vi "Rcv Cmd.vi"(8 "error in":errorcluster, 11 "nPAS in":refnum<class "nPAS.lvclass">) -> (0 "error out":errorcluster, 3 "nPAS out":refnum<class "nPAS.lvclass">)   [LabVIEW 2015, in "nPAS.lvclass"]
doc: "This function is abstract and the child must overide it. This function should provide a means by which the user may interact with the PAS."
uses:
  nPAS.lvclass
  Session/Raw FPGA/FPGA Session.lvclass
  nPAS.lvclass/nPAS.ctl
  Session/Raw FPGA/FPGA Session.lvclass/FPGA Session.ctl
  FPGA/fpga dio enum.ctl
  Reusable/PAS/Main/PAS.lvclass/PAS.ctl
  Reusable/Instrument/state.ctl
  Reusable/PAS/Main/Write Chirp.vi
  Session/Raw FPGA/Read FPGA Ref.vi
  <vilib>/Utility/error.llb/Error Cluster From Error Code.vi
  <vilib>/rvi/errors/niLvFpgaAdjustHostInterfaceError.vi
  Reusable/PAS/Main/Set Speaker Switch.vi
  FPGA Ref.ctl
  <vilib>/rvi/interface/nirviReadWriteControl/nirviReadWriteControl.xnode
  FPGA Bitfiles/NickIO.lvbitx
  <vilib>/rvi/interface/nirviMethod/nirviMethod.xnode
  FPGA/PAS Modulation.ctl
  Reusable/Instrument/Instrument.lvclass
  NiFpgaLv.dll
  <vilib>/rvi/errors/niLvFpgaMergeErrorWithErrorCode.vi
  <vilib>/FPGAPlugInAG/cRIO-9081/niLvFpga_WriteFifo_cRIO-9081.vi
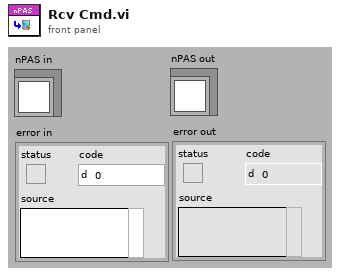
[diagram p1: front panel]
types:
  T1 = typedef "fpga dio enum.ctl" = enum16{"uv.ctl_1", "uv.ctl_2", "uv.enable", "pas.las_enable", "pas.speaker", "compressor", "vacuum", "sol.o3_add", "sol.scubber_test", "sol.pmeas1", "sol.pmeas2", "filt.hb_ctl_1", "filt.hb_ctl_2", "crd.las_enable"}
  T2 = typedef "Instrument.lvclass/state.ctl" = enum8{"Configure", "Acquire", "Wait", "Quit", "Handle Error", "NOOP"}
  T3 = typedef "Session - Root.lvclass/Session Handle.ctl" = refnum<data-value>
  T4 = typedef "FPGA Ref.ctl" = refnum<k20>
  T5 = cluster{"Array of Int16[0]":i16, "Array of Int16[1]":i16}
  T6 = typedef "PAS Modulation.ctl" = cluster{"f0":fxp<+,32,0>, "Mod":u8, "Vscale":fxp<+,32,0>, "Offset":i16}
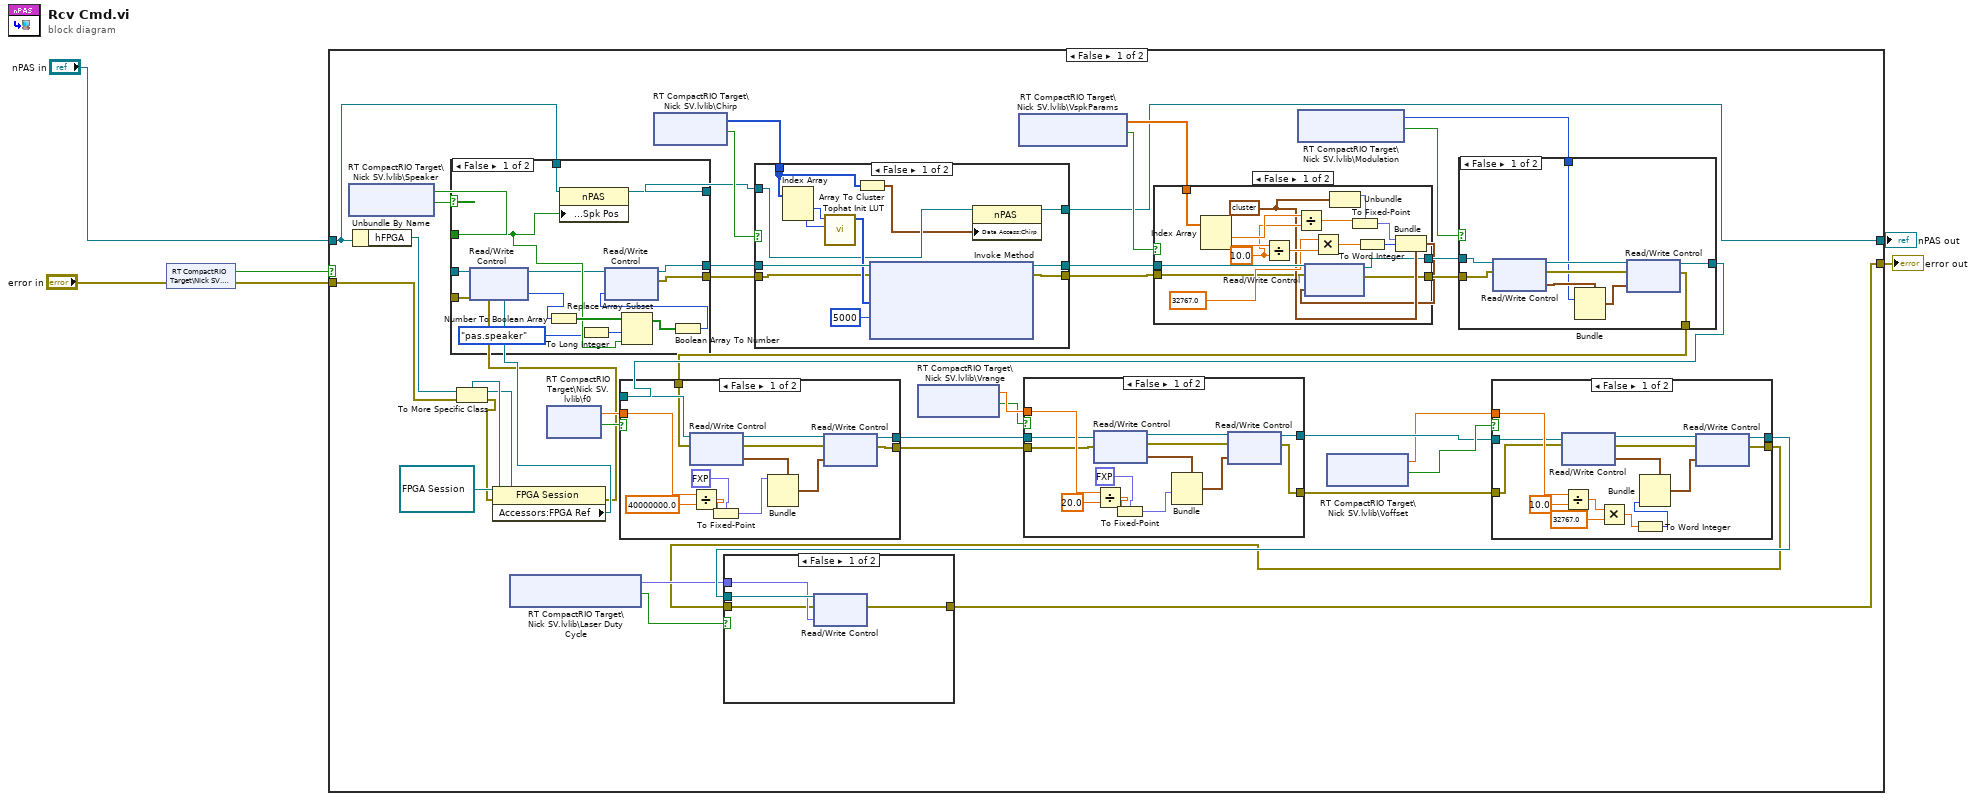
[diagram p0: block diagram]
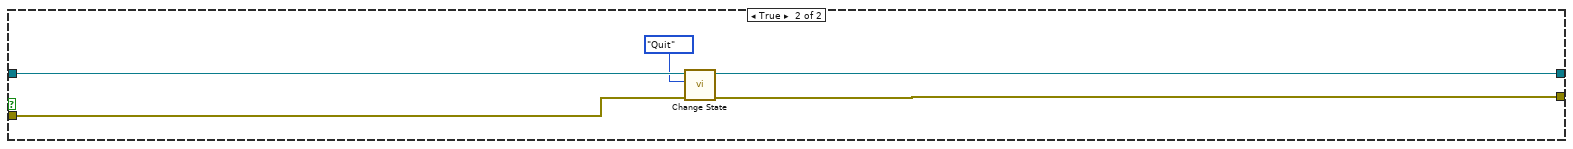
[diagram p10: hidden frame]
diagram:
  n1 = shared-variable "RT CompactRIO Target\\Nick SV.lvlib\\Stop"(error in="error in") -> (w5:bool, error out=w2:errorcluster)
  n2 = case shown="False" w5 {
    tunnel: "nPAS in" -> [w9 w165]
    tunnel: [w7 w164] -> w3
    tunnel: w2 -> [w14 w162]
    tunnel: [w18 w161] -> w1
    frame False {
      n3 = shared-variable "RT CompactRIO Target\\Nick SV.lvlib\\Speaker"() -> (w46:bool, w47:bool)  [unwired: 2 in, 1 out]
      n4 = Unbundle By Name(w9) -> ("hFPGA"=w16:T3)
      n5 = To More Specific Class(target class=refnum<data-value> refnum ("hFPGA"), reference=w16, error in=w14) -> (specific class reference=w13:refnum<data-value>, error out=w12:errorcluster)
      n6 = property class="FPGA Session"(reference=w13, error in=w12) -> (error out=w10:errorcluster, "Accessors:FPGA Ref"=w11:T4)  [unwired: 1 out]
      n7 = case shown="False" w47 {
        tunnel: w46 -> [w149 _]
        tunnel: w11 -> [w153 w160]
        tunnel: [w157 w160] -> w43
        tunnel: [w156 w159] -> w28
        tunnel: w10 -> [w152 w159]
        tunnel: w9 -> [w155 w158]
        tunnel: [w154 w158] -> w8
        frame False {
          n8 = xnode "Read/Write Control"("FPGA VI Reference In"=w153, "error in"=w152) -> ("FPGA VI Reference Out"=w147:T4, "DO Out"=w151:u16)  [unwired: 1 out]
          n9 = Number To Boolean Array(number=w151) -> (Boolean array=w150:bool[])
          n10 = property class="nPAS"(reference=w155, "Data Access:Spk Pos"=w149) -> (reference out=w154:refnum<class "nPAS.lvclass">)  [unwired: 1 in, 1 out]
          n11 = To Long Integer(number=fpga_dio_enum."pas.speaker" ("fpga dio")) -> (32bit integer=w146:i32)
          n12 = Replace Array Subset(array=w150, new element=w149, index=w146) -> (w148:bool[])
          n13 = Boolean Array To Number(Boolean array=w148) -> (number=w144:u16)
          n14 = xnode "Read/Write Control"("FPGA VI Reference In"=w147, "DO In"=w144) -> ("FPGA VI Reference Out"=w157:T4, "error out"=w156:errorcluster)  [unwired: 1 in]
        }
        frame True {
        }
      }
      n15 = shared-variable "RT CompactRIO Target\\Nick SV.lvlib\\Laser Duty Cycle"() -> (w20:fxp<+,32,0>, w22:bool)  [unwired: 2 in, 1 out]
      n16 = shared-variable "RT CompactRIO Target\\Nick SV.lvlib\\f0"() -> (w35:dbl, w36:bool)  [unwired: 2 in, 1 out]
      n17 = shared-variable "RT CompactRIO Target\\Nick SV.lvlib\\Chirp"() -> (w44:i16[], w45:bool)  [unwired: 2 in, 1 out]
      n18 = case shown="False" w45 {
        tunnel: w44 -> [w130 _]
        tunnel: w43 -> [w138 w143]
        tunnel: [w135 w143] -> w41
        tunnel: w28 -> [w134 w142]
        tunnel: [w133 w142] -> w27
        tunnel: w8 -> [w132 w141]
        tunnel: [w131 w141] -> w7
        frame False {
          n19 = Index Array(array=w130) -> (element #1=w140:i16, element #2=w139:i16)  [unwired: 2 in]
          n20 = call "Tophat Init LUT.vi"("Df"=w139, "f0"=w140) -> ("Init Data Out"=w137:i16[])  [unwired: 7 in]
          n21 = Array To Cluster(array=w130) -> (cluster=w129:T5)
          n22 = xnode "Invoke Method"("FPGA VI Reference In"=w138, "error in"=w134, "Data"=w137, "Timeout (ms)"=5000) -> ("FPGA VI Reference Out"=w135:T4, "error out"=w133:errorcluster)  [unwired: 1 out]
          n23 = property class="nPAS"(reference=w132, "Data Access:Chirp"=w129) -> (reference out=w131:refnum<class "nPAS.lvclass">)  [unwired: 1 in, 1 out]
        }
        frame True {
        }
      }
      n24 = shared-variable "RT CompactRIO Target\\Nick SV.lvlib\\Vrange"() -> (w32:dbl, w17:bool)  [unwired: 2 in, 1 out]
      n25 = shared-variable "RT CompactRIO Target\\Nick SV.lvlib\\VspkParams"() -> (w40:sgl[], w42:bool)  [unwired: 2 in, 1 out]
      n26 = case shown="False" w42 {
        tunnel: w41 -> [w126 w128]
        tunnel: w40 -> [w125 _]
        tunnel: [w112 w128] -> w38
        tunnel: w27 -> [w111 w127]
        tunnel: [w110 w127] -> w26
        frame False {
          w119 = sgl 10.0 ("y")
          w116 = cluster{"Vscale":fxp<+,32,0>, "Offset":i16} {"Vscale"=0.0, "Offset"=0} ("Speaker")
          n27 = Index Array(array=w125) -> (element #1=w120:sgl, element #2=w124:sgl)  [unwired: 2 in]
          n28 = Divide(x=w124, y=w119) -> (x/y=w123:sgl)
          n29 = Divide(x=w120, y=w119) -> (x/y=w118:sgl)
          n30 = Multiply(x=sgl 32767.0, y=w123) -> (x*y=w121:sgl)
          n31 = Unbundle(w116) -> ("Vscale"=w117:fxp<+,32,0>)  [unwired: 1 out]
          n32 = To Fixed-Point(fixed-point type=w117, number=w118) -> (fixed-point=w115:fxp<+,32,0>)
          n33 = To Word Integer(number=w121) -> (16bit integer=w114:i16)
          n34 = Bundle(cluster=w116, "Vscale"=w115, "Offset"=w114) -> (w113:cluster{"Vscale":fxp<+,32,0>, "Offset":i16})
          n35 = xnode "Read/Write Control"("FPGA VI Reference In"=w126, "error in"=w111, "Speaker"=w113) -> ("FPGA VI Reference Out"=w112:T4, "error out"=w110:errorcluster)
        }
        frame True {
        }
      }
      n36 = shared-variable "RT CompactRIO Target\\Nick SV.lvlib\\Modulation"() -> (w37:u8, w39:bool)  [unwired: 2 in, 1 out]
      n37 = shared-variable "RT CompactRIO Target\\Nick SV.lvlib\\Voffset"() -> (w29:dbl, w31:bool)  [unwired: 2 in, 1 out]
      n38 = case shown="False" w39 {
        tunnel: w38 -> [w107 w109]
        tunnel: w37 -> [w99 _]
        tunnel: [w103 w109] -> w34
        tunnel: w26 -> [w102 w108]
        tunnel: [w100 w108] -> w25
        frame False {
          n39 = xnode "Read/Write Control"("FPGA VI Reference In"=w107, "error in"=w102) -> ("FPGA VI Reference Out"=w105:T4, "error out"=w101:errorcluster, "Wave"=w106:T6)
          n40 = Bundle(cluster=w106, "Mod"=w99) -> (w104:T6)  [unwired: 3 in]
          n41 = xnode "Read/Write Control"("FPGA VI Reference In"=w105, "error in"=w101, "Wave"=w104) -> ("FPGA VI Reference Out"=w103:T4, "error out"=w100:errorcluster)
        }
        frame True {
        }
      }
      n42 = case shown="False" w36 {
        tunnel: w35 -> [w94 _]
        tunnel: w34 -> [w88 w98]
        tunnel: [w87 w98] -> w33
        tunnel: w25 -> [w86 w97]
        tunnel: [w84 w97] -> w24
        frame False {
          n43 = xnode "Read/Write Control"("FPGA VI Reference In"=w88, "error in"=w86) -> ("FPGA VI Reference Out"=w96:T4, "error out"=w85:errorcluster, "Wave"=w95:T6)
          n44 = Divide(x=w94, y=40000000.0) -> (x/y=w92:dbl)
          n45 = To Fixed-Point(fixed-point type=fxp<+,32,0> 0.0 ("f0"), number=w92) -> (fixed-point=w90:fxp<+,32,0>)
          n46 = Bundle(cluster=w95, "f0"=w90) -> (w89:T6)  [unwired: 3 in]
          n47 = xnode "Read/Write Control"("FPGA VI Reference In"=w96, "error in"=w85, "Wave"=w89) -> ("FPGA VI Reference Out"=w87:T4, "error out"=w84:errorcluster)
        }
        frame True {
        }
      }
      n48 = case shown="False" w17 {
        tunnel: w32 -> [w79 _]
        tunnel: w33 -> [w74 w83]
        tunnel: [w73 w83] -> w30
        tunnel: w24 -> [w71 w82]
        tunnel: [w69 w82] -> w23
        frame False {
          n49 = xnode "Read/Write Control"("FPGA VI Reference In"=w74, "error in"=w71) -> ("FPGA VI Reference Out"=w81:T4, "error out"=w70:errorcluster, "Wave"=w80:T6)
          n50 = Divide(x=w79, y=20.0) -> (x/y=w77:dbl)
          n51 = To Fixed-Point(fixed-point type=fxp<+,32,0> 0.0 ("f0"), number=w77) -> (fixed-point=w72:fxp<+,32,0>)
          n52 = Bundle(cluster=w80, "Vscale"=w72) -> (w75:T6)  [unwired: 3 in]
          n53 = xnode "Read/Write Control"("FPGA VI Reference In"=w81, "error in"=w70, "Wave"=w75) -> ("FPGA VI Reference Out"=w73:T4, "error out"=w69:errorcluster)
        }
        frame True {
        }
      }
      n54 = case shown="False" w31 {
        tunnel: w29 -> [w64 _]
        tunnel: w30 -> [w61 w68]
        tunnel: [w60 w68] -> w21
        tunnel: w23 -> [w55 w67]
        tunnel: [w53 w67] -> w19
        frame False {
          n55 = xnode "Read/Write Control"("FPGA VI Reference In"=w61, "error in"=w55) -> ("FPGA VI Reference Out"=w66:T4, "error out"=w54:errorcluster, "Wave"=w65:T6)
          n56 = Divide(x=w64, y=10.0) -> (x/y=w59:dbl)
          n57 = Multiply(x=w59, y=32767.0) -> (x*y=w57:dbl)
          n58 = To Word Integer(number=w57) -> (16bit integer=w56:i16)
          n59 = Bundle(cluster=w65, "Offset"=w56) -> (w62:T6)  [unwired: 3 in]
          n60 = xnode "Read/Write Control"("FPGA VI Reference In"=w66, "error in"=w54, "Wave"=w62) -> ("FPGA VI Reference Out"=w60:T4, "error out"=w53:errorcluster)
        }
        frame True {
        }
      }
      n61 = case shown="False" w22 {
        tunnel: w21 -> [w51 _]
        tunnel: w20 -> [w50 _]
        tunnel: w19 -> [w49 w52]
        tunnel: [w48 w52] -> w18
        frame False {
          n62 = xnode "Read/Write Control"("FPGA VI Reference In"=w51, "error in"=w49, "pDC"=w50) -> ("error out"=w48:errorcluster)  [unwired: 1 out]
        }
        frame True {
        }
      }
    }
    frame True {
      n63 = call "Change State.vi"("error in"=w162, "instr state"=state."Quit", "Instrument in"=w165) -> ("error out"=w161:errorcluster, "Instrument out"=w164:refnum<class "nPAS.lvclass">)  [unwired: 7 in]
    }
  }
  "error out" <- w1
  "nPAS out" <- w3
